vi "Extract Complete Message.vi"(8 "Error in (no error)":errorcluster, 10 "Text to prepend to messages":string, 11 "String of Instrument Messages":string) -> (0 "Error out":errorcluster, 2 "Remaining String":string, 3 "Ocean Server Sentences":string[](array[string]))   [LabVIEW 2011, in "Ocean Server OS4000.lvlib"]
doc: "Parses the entire string of sentence from the instrument to a complete sentence. Any partial messages found at the end of the string are returned in <b>Remaining String</b>.\n\n<b>Note:</b> If the string of sentence from instrument does not pass checksum then it will be discarded."
uses:
  Ocean Server OS4000.lvlib
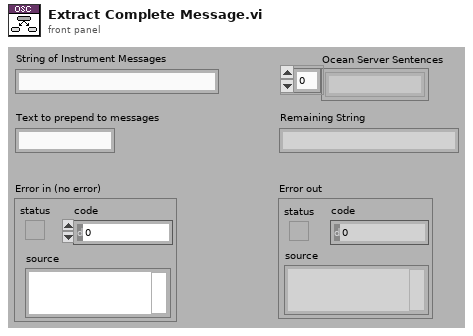
[diagram p1: front panel]
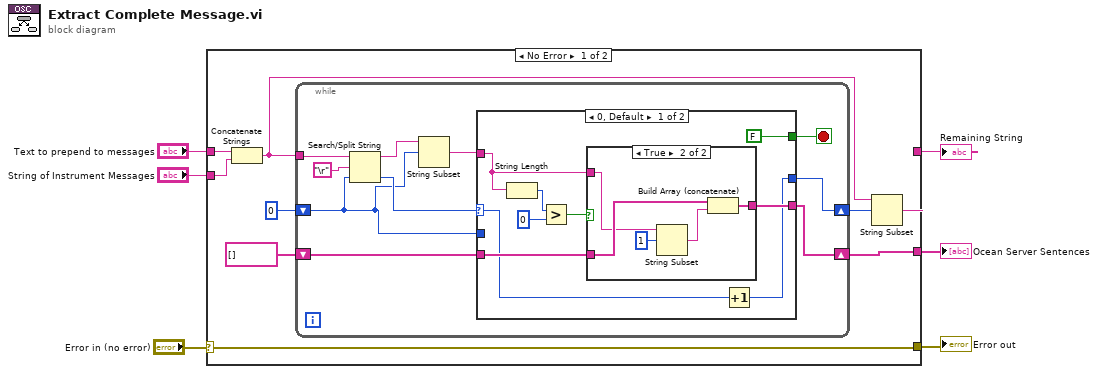
[diagram p0: block diagram]
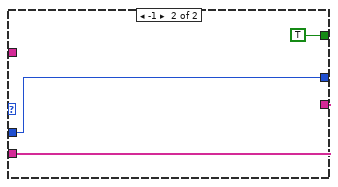
[diagram p3: hidden frame]
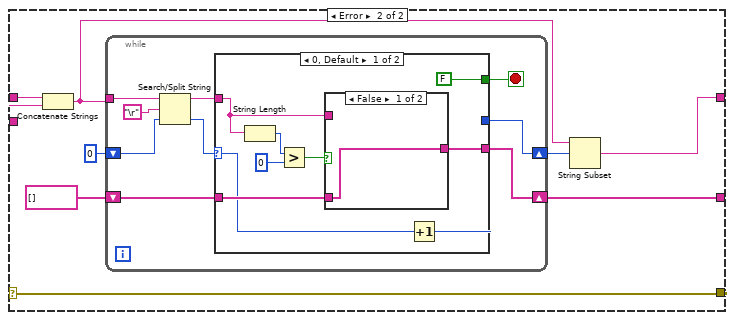
[diagram p4: hidden frame]
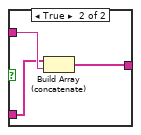
[diagram p5: hidden frame]
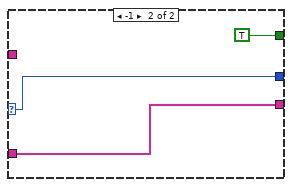
[diagram p6: hidden frame]
diagram:
  n1 = case shown="No Error" "Error in (no error)" {
    selector: "Error in (no error)" -> [w15 w52]
    tunnel: [w15 w52] -> w6
    tunnel: "String of Instrument Messages" -> [w14 w46]
    tunnel: "Text to prepend to messages" -> [w13 w47]
    tunnel: [w8 w45] -> w3
    tunnel: [w7 w44] -> w1
    frame No Error {
      n2 = Concatenate Strings(w13, w14) -> (w10:string)
      n3 = while {
        tunnel: w10 -> [w25]
        shift-right: [w21] -> w7
        shift-left: string[] [] ("array") -> [w22]
        shift-right: [w19] -> w9
        shift-left: 0 -> [w17]
        stop <- w20 stop-if-true
        n4 = Search/Split String(string=w25, search string/char (-)="\r", offset (0)=w17) -> (substring before match=w16:string, offset of match=w23:i32)  [unwired: 1 out]
        n5 = String Subset(string=w16, offset (0)=w17) -> (substring=w18:string)  [unwired: 1 in]
        n6 = case shown="0, Default" w23 {
          selector: w23 -> [w28 _]
          tunnel: w18 -> [w31 _]
          tunnel: w22 -> [w30 w42]
          tunnel: [w29 w42] -> w21
          tunnel: [FALSE TRUE] -> w20
          tunnel: [w27 w41] -> w19
          tunnel: w17 -> [_ w41]
          frame 0, Default {
            n7 = String Length(string=w31) -> (length=w33:i32)
            n8 = Greater?(x=w33, y=0) -> (0:w34:bool)
            n9 = case shown="True" w34 {
              tunnel: w31 -> [_ w37]
              tunnel: w30 -> [w35 w40]
              tunnel: [w35 w39] -> w29
              frame False {
              }
              frame True {
                n10 = String Subset(string=w37, offset (0)=1) -> (substring=w36:string)  [unwired: 1 in]
                n11 = Build Array (concatenate)(w40, w36) -> (w39:string[])
              }
            }
            n12 = Increment(x=w28) -> (x+1=w27:i32)
          }
          frame -1 {
          }
        }
      }
      n13 = String Subset(string=w10, offset (0)=w9) -> (substring=w8:string)  [unwired: 1 in]
    }
    frame Error {
      n14 = Concatenate Strings(w47, w46) -> (w49:string)
      n15 = while {
        tunnel: w49 -> [w61]
        shift-right: [w56] -> w44
        shift-left: string[] [] ("array") -> [w57]
        shift-right: [w54] -> w48
        shift-left: 0 -> [w53]
        stop <- w55 stop-if-true
        n16 = Search/Split String(string=w61, search string/char (-)="\r", offset (0)=w53) -> (substring before match=w58:string, offset of match=w59:i32)  [unwired: 1 out]
        n17 = case shown="0, Default" w59 {
          selector: w59 -> [w64 w75]
          tunnel: w58 -> [w67 _]
          tunnel: w57 -> [w66 w76]
          tunnel: [w65 w76] -> w56
          tunnel: [FALSE TRUE] -> w55
          tunnel: [w63 w75] -> w54
          frame 0, Default {
            n18 = String Length(string=w67) -> (length=w69:i32)
            n19 = Greater?(x=w69, y=0) -> (0:w70:bool)
            n20 = case shown="False" w70 {
              tunnel: w67 -> [_ w74]
              tunnel: w66 -> [w71 w73]
              tunnel: [w71 w72] -> w65
              frame False {
              }
              frame True {
                n21 = Build Array (concatenate)(w73, w74) -> (w72:string[])
              }
            }
            n22 = Increment(x=w64) -> (x+1=w63:i32)
          }
          frame -1 {
          }
        }
      }
      n23 = String Subset(string=w49, offset (0)=w48) -> (substring=w45:string)  [unwired: 1 in]
    }
  }
  "Remaining String" <- w3
  "Error out" <- w6
  "Ocean Server Sentences" <- w1
